vi "Tosca-Purge Locomotion Data.vi"(0 "Path":path, 11 "error in (no error)":errorcluster) -> (15 "error out":errorcluster)   [LabVIEW 2020]
uses:
  epl-vi-lib/TCP VIs/TCP Params.ctl
  Tosca-Globals.vi
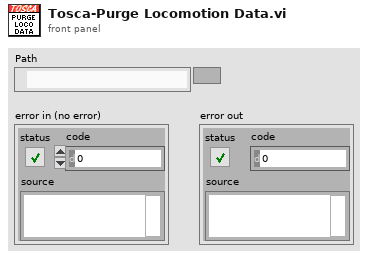
[diagram p1: front panel]
types:
  T1 = typedef "TCP Params.ctl" = cluster{"IP Address":string, "Port":i32}
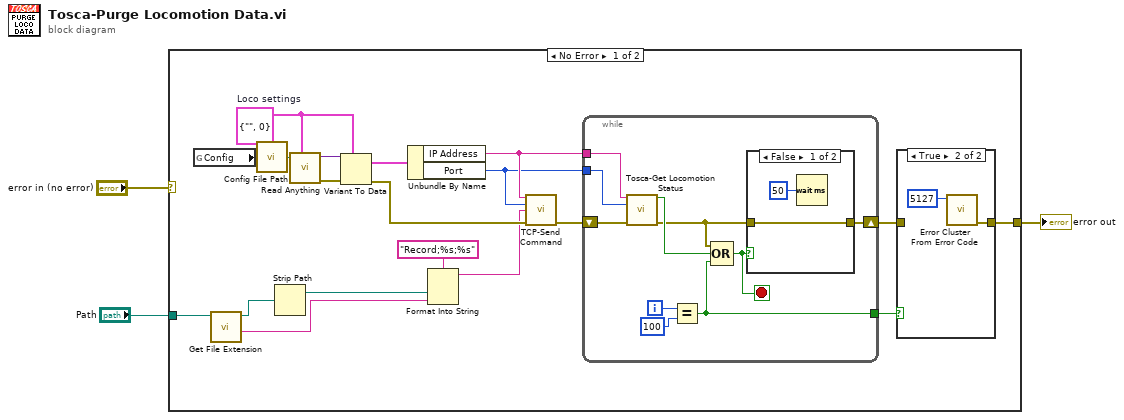
[diagram p0: block diagram]
diagram:
  n1 = case shown="No Error" "error in (no error)" {
    selector: "error in (no error)" -> [_ w39]
    tunnel: [w8 w39] -> w2
    tunnel: "Path" -> [w16 _]
    frame No Error {
      w21 = T1 {"IP Address"="", "Port"=0}  # Loco settings
      n2 = global read "Tosca-Globals.vi" "Config"() -> (w4:string)
      n3 = call <vilib>:"Get File Extension.vi"("file"=w16) -> ("filename without extension"=w12:string, "dup file"=w14:path)  [unwired: 6 in, 3 out]
      n4 = call "Config File Path.vi"("AppName"=w4) -> ("Default config file name"=w22:path)
      n5 = Strip Path(path=w14) -> (stripped path=w13:path)  [unwired: 1 out]
      n6 = call "Read Anything.vi"("Type of Anything"=w21, "Path (dialog)"=w22) -> ("Error Out"=w19:errorcluster, "Anything"=w20:variant)  [unwired: 7 in, 1 out]
      n7 = Variant To Data(error in=w19, type=w21, Variant=w20) -> (data=w18:T1, error out=w17:errorcluster)
      n8 = Unbundle By Name(w18) -> ("IP Address"=w11:string, "Port"=w10:i32)
      n9 = Format Into String(format string="Record;%s;%s", w13, w12) -> (resulting string=w5:string)  [unwired: 2 in, 1 out]
      n10 = call "TCP-Send Command.vi"("PXI Address"=w11, "Port"=w10, "Command"=w5, "error in (no error)"=w17) -> ("error out"=w9:errorcluster)  [unwired: 11 in]
      n11 = while {
        tunnel: w11 -> [w32]
        tunnel: w10 -> [w31]
        shift-right: [w27] -> w6
        shift-left: w9 -> [w30]
        tunnel: [w24] -> w7
        i -> [w26]
        stop <- w25 stop-if-true
        n12 = call "Tosca-Get Locomotion Status.vi"("IP Address"=w32, "Port"=w31, "error in (no error)"=w30) -> ("Recording"=w29:bool, "error out"=w28:errorcluster)  [unwired: 11 in]
        n13 = Equal?(x=w26, y=100) -> (x = y?=w24:bool)
        n14 = Compound Arithmetic op=OR(w28, w29, w24) -> (w25:bool)
        n15 = case shown="False" w25 {
          tunnel: w28 -> [w33 w35]
          tunnel: [w33 w35] -> w27
          frame False {
            n16 = Wait (ms)(milliseconds to wait=u32 50) -> ()  [unwired: 1 out]
          }
          frame True {
          }
        }
      }
      n17 = case shown="True" w7 {
        tunnel: w6 -> [w36 _]
        tunnel: [w36 w38] -> w8
        frame False {
        }
        frame True {
          n18 = call <vilib>:"Error Cluster From Error Code.vi"("error code (0)"=5127) -> ("error out"=w38:errorcluster)  [unwired: 8 in]
        }
      }
    }
    frame Error {
    }
  }
  "error out" <- w2
